vi "编码器角度位置测量_单点_滤波_反转.vi"() -> ()   [LabVIEW 2013]
uses:
  <userlib>/ArtDAQ/_SubVI/ArtDAQ_CreateCIAngEncoderChan.vi
  <userlib>/ArtDAQ/_SubVI/ArtDAQ_Read Counter DBL 1Samp.vi
panel:
  in  "Aux最小滤波脉宽(s)":dbl
  in  "Gate最小滤波脉宽(s)":dbl
  in  "Src最小滤波脉宽(s)":dbl
  in  "启用Z反转":bool
  in  "启用B反转":bool
  in  "启用A反转":bool
  in  "Z索引相位":i32(ring)=10040 items=["A高B高"=10040, "A高B低"=10041, "A低B高"=10042, "A低B低"=10043]
  in  "解码类型":i32(ring)=10090 items=["X1"=10090, "X2"=10091, "X4"=10092, "双脉冲"=10313]
  out "数据(度)":dbl
  in  "初始角度":dbl
  in  "脉冲/转":u32=2000
  in  "Z索引值":dbl
  in  "启用Z索引":bool
  in  "Stop":bool
  in  "计数器":string="Dev1/ctr0"
  out "错误输出":errorcluster
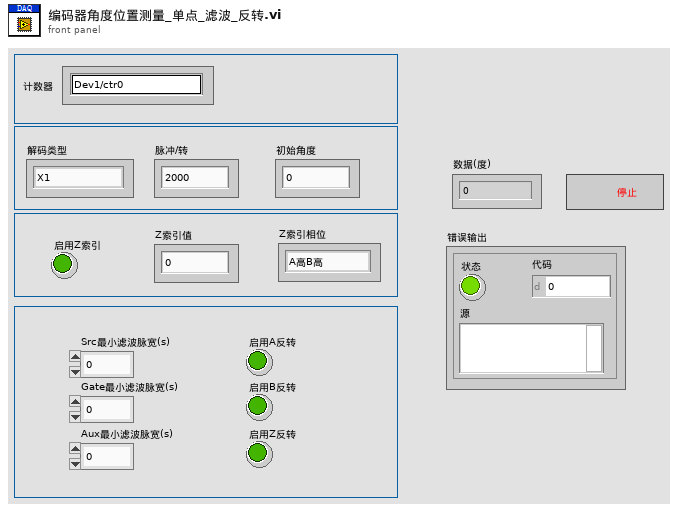
[diagram p1: front panel]
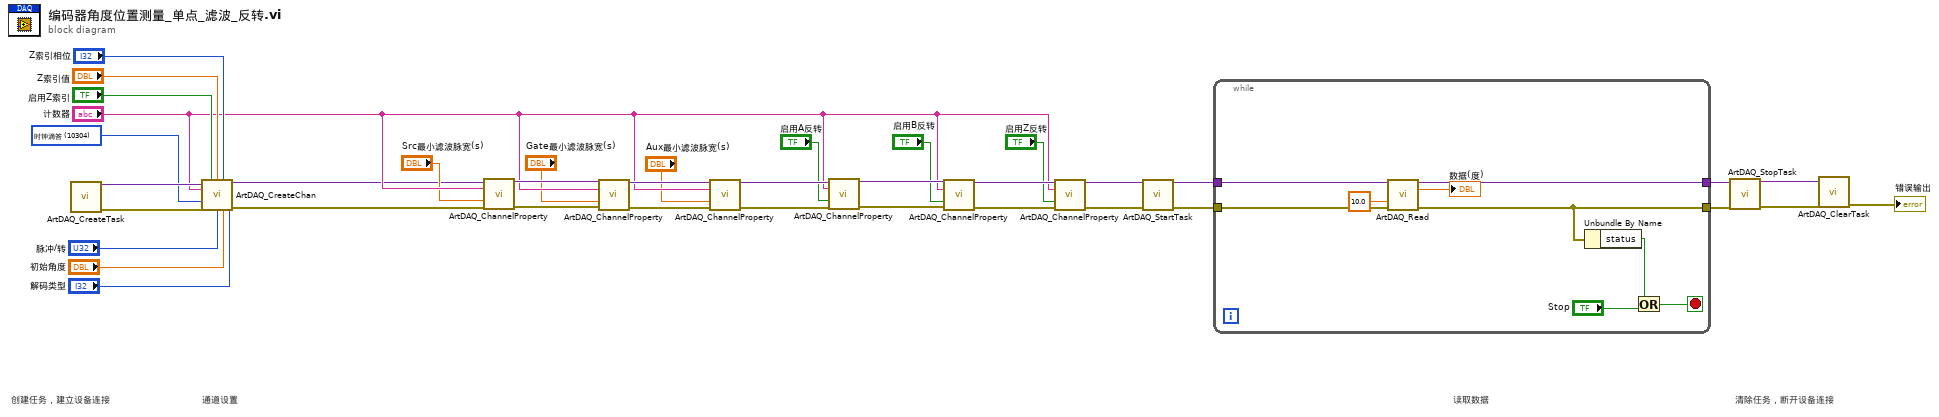
[diagram p0: block diagram]
diagram:
  w24 = 10304 items=["度"=10146, "弧度"=10273, "时钟滴答"=10304, "来自自定义换算"=10065] ("单位")
  # "清除任务，断开设备连接"
  # "读取数据"
  # "通道设置"
  # "创建任务，建立设备连接"
  n1 = call <userlib>:"ArtDAQ_CreateTask.vi"() -> ("任务句柄"=w37:variant, "错误输出"=w36:errorcluster)  [unwired: 14 in]
  n2 = call-poly <userlib>:"ArtDAQ_CreateChan.vi"("任务句柄"=w37, "启用Z索引"="启用Z索引", "Z索引值"="Z索引值", "Z索引相位"="Z索引相位", "计数器"="计数器", "解码类型"="解码类型", "单位"=w24, "错误输入"=w36, "脉冲每转"="脉冲/转", "初始角"="初始角度") -> ("任务句柄"=w5:variant, "错误输出"=w4:errorcluster)  [unwired: 4 in]
  n3 = call-poly <userlib>:"ArtDAQ_ChannelProperty.vi"("任务句柄"=w5, "计数器通道"="计数器", "脉宽(s)"="Src最小滤波脉宽(s)", "ErrorInput"=w4) -> ("任务句柄"=w23:variant, "ErrorOutput"=w18:errorcluster)  [unwired: 10 in]
  n4 = call-poly <userlib>:"ArtDAQ_ChannelProperty.vi"("任务句柄"=w23, "计数器通道"="计数器", "脉宽(s)"="Gate最小滤波脉宽(s)", "ErrorInput"=w18) -> ("任务句柄"=w22:variant, "ErrorOutput"=w17:errorcluster)  [unwired: 10 in]
  n5 = call-poly <userlib>:"ArtDAQ_ChannelProperty.vi"("任务句柄"=w22, "计数器通道"="计数器", "脉宽(s)"="Aux最小滤波脉宽(s)", "ErrorInput"=w17) -> ("任务句柄"=w21:variant, "ErrorOutput"=w16:errorcluster)  [unwired: 10 in]
  n6 = call-poly <userlib>:"ArtDAQ_ChannelProperty.vi"("任务句柄"=w21, "计数器通道"="计数器", "是否取反？(s)"="启用A反转", "ErrorInput"=w16) -> ("任务句柄"=w20:variant, "ErrorOutput"=w15:errorcluster)  [unwired: 10 in]
  n7 = call-poly <userlib>:"ArtDAQ_ChannelProperty.vi"("任务句柄"=w20, "计数器通道"="计数器", "是否取反？(s)"="启用B反转", "ErrorInput"=w15) -> ("任务句柄"=w19:variant, "ErrorOutput"=w14:errorcluster)  [unwired: 10 in]
  n8 = call-poly <userlib>:"ArtDAQ_ChannelProperty.vi"("任务句柄"=w19, "计数器通道"="计数器", "是否取反？(s)"="启用Z反转", "ErrorInput"=w14) -> ("任务句柄"=w1:variant, "ErrorOutput"=w3:errorcluster)  [unwired: 10 in]
  n9 = call <userlib>:"ArtDAQ_StartTask.vi"("任务句柄"=w1, "错误输入"=w3) -> ("任务句柄"=w6:variant, "错误输出"=w2:errorcluster)  [unwired: 12 in]
  n10 = while {
    tunnel: [w46] -> w35
    tunnel: [w45] -> w33
    tunnel: w6 -> [w44]
    tunnel: w2 -> [w43]
    stop <- w40 stop-if-true
    n11 = call-poly <userlib>:"ArtDAQ_Read.vi"("任务句柄"=w44, "超时s"=10.0 ("Timeout"), "错误输入"=w43) -> ("任务句柄"=w46:variant, "数据"=→"数据(度)":dbl, "错误输出"=w45:errorcluster)  [unwired: 10 in]
    n12 = Unbundle By Name(w45) -> ("status"=w42:bool)
    n13 = Or(x=w42, y="Stop") -> (x .or. y?=w40:bool)
  }
  n14 = call <userlib>:"ArtDAQ_StopTask.vi"("任务句柄"=w35, "错误输入"=w33) -> ("任务句柄"=w34:variant, "错误输出"=w32:errorcluster)  [unwired: 12 in]
  n15 = call <userlib>:"ArtDAQ_ClearTask.vi"("任务句柄"=w34, "错误输入"=w32) -> ("错误输出"=→"错误输出":errorcluster)  [unwired: 13 in]
